vi "Page_Exclusions_Initialize.vi"(8 "error in (no error)":errorcluster, 9 "ctlReferences":T1, 11 "AB_Targetfile in":refnum<class "AB_Targetfile.lvclass">) -> (0 "error out":errorcluster, 3 "AB_Targetfile out":refnum<class "AB_Targetfile.lvclass">)   [LabVIEW 2020, in "AB_Targetfile.lvclass"]
uses:
  <vilib>/AppBuilder/AB_Classes/TargetFile/AB_Targetfile.lvclass
  <resource>/Framework/Providers/Builds/AppBuilder/AB_UI_Page_Exclusions_References.ctl
  <vilib>/AppBuilder/AB_Classes/Build/AB_Build.lvclass
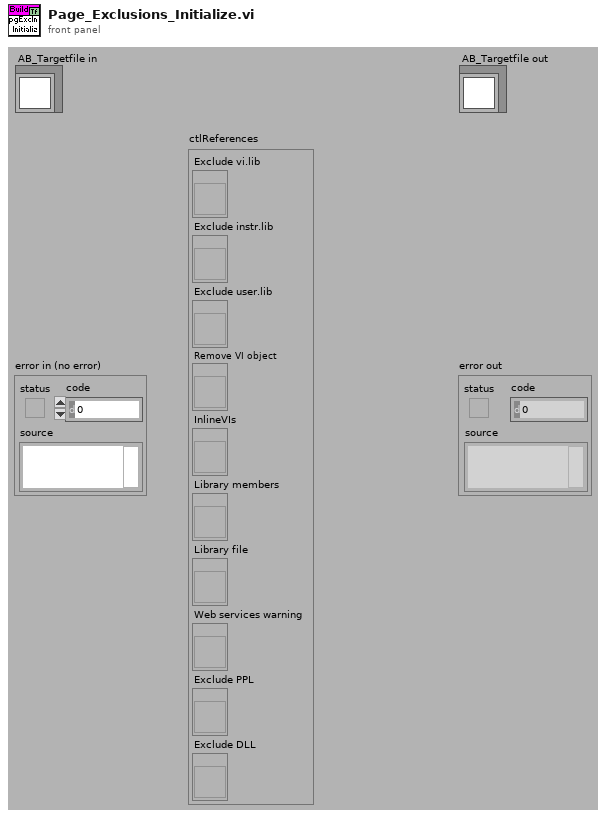
[diagram p1: front panel]
types:
  T1 = typedef "AB_UI_Page_Exclusions_References.ctl" = cluster{"Exclude vi.lib":refnum<vi>, "Exclude instr.lib":refnum<vi>, "Exclude user.lib":refnum<vi>, "Remove VI object":refnum<vi>, "InlineVIs":refnum<vi>, "Library members":refnum<vi>, "Library file":refnum<vi>, "Web services warning":refnum<vi>, "Exclude PPL":refnum<vi>, "Exclude DLL":refnum<vi>}
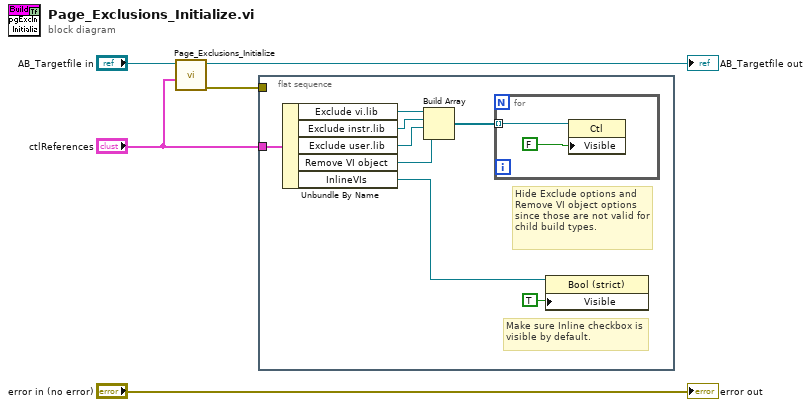
[diagram p0: block diagram]
diagram:
  n1 = call-parent "Page_Exclusions_Initialize.vi"("ctlReferences"="ctlReferences", "AB_Build in"="AB_Targetfile in") -> ("error out"=w1:errorcluster, "AB_Build out"=→"AB_Targetfile out":refnum<class "AB_Targetfile.lvclass">)  [unwired: 8 in]
  n2 = flat-sequence {
    tunnel: "ctlReferences" -> [w6]
    tunnel: w1 -> [_]
    frame #0 {
      # "Make sure Inline checkbox is visible by default."
      # "Hide Exclude options and Remove VI object options since those are not valid for child build types."
      n3 = Unbundle By Name(w6) -> ("Exclude vi.lib"=w13:refnum<vi>, "Exclude instr.lib"=w12:refnum<vi>, "Exclude user.lib"=w11:refnum<vi>, "Remove VI object"=w10:refnum<vi>, "InlineVIs"=w7:refnum<vi>)
      n4 = Build Array(w13, w12, w11, w10) -> (w9:refnum<vi>[])
      n5 = for {
        tunnel: w9 -> [w15] mode=indexing
        n6 = property class="Ctl"(reference=w15, "Visible"=FALSE) -> ()  [unwired: 1 in, 2 out]
      }
      n7 = property class="Bool (strict)"(reference=w7, "Visible"=TRUE) -> ()  [unwired: 1 in, 2 out]
    }
  }
  "error out" <- "error in (no error)"
